vi "GetHelp.vi"(11 "CoreOperation in":refnum<class "CoreOperation.lvclass">) -> (2 "Help":string, 3 "CoreOperation out":refnum<class "CoreOperation.lvclass">)   [LabVIEW 2014, in "CoreOperation.lvclass"]
uses:
  CoreOperation.lvclass
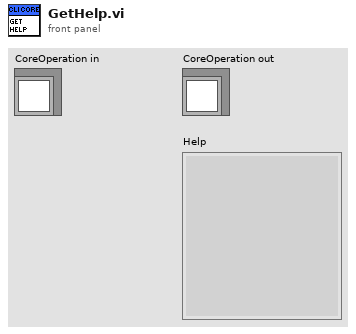
[diagram p1: front panel]
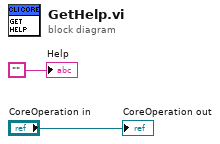
[diagram p0: block diagram]
diagram:
  "CoreOperation out" <- "CoreOperation in"
  "Help" <- ""
